vi "Teleop.vi"(10 "Match Info":T1={"Autonomous Elapsed Seconds"=0.0, "TeleOp Elapsed Seconds"=0.0, "Disabled Elapsed Seconds"=0.0, "Visited Autonomous"=FALSE, "Visited TeleOp"=FALSE, "Visited Disabled"=FALSE, "Autonomous Settings"={"Autonomous Style"=enum."Independent", "VI Refnum"=refnum}}, 11 "Call Context":T2) -> ()   [LabVIEW 2015]
doc: "This VI is called for each TeleOp packet received from the DS where the robot is not disabled. It is often used to read from the joysticks and update I/O or to update setpoints for timed control loops. It should complete and return within 20 milliseconds or it may miss DS packets."
uses:
  <vilib>/Rock Robotics/WPI/DriverStation/WPI_DriverStationDerivedRobotMode.ctl
  <vilib>/Rock Robotics/WPI/DriverStation/WPI_DriverStationMatch Info.ctl
  <vilib>/Rock Robotics/WPI/Solenoid/WPI_SolenoidValue.ctl
  <vilib>/Rock Robotics/WPI/Utilities/WPI_GetSetVariantRefNum.vi
  <vilib>/Rock Robotics/Network Tables/NT Read Boolean.vi
  <vilib>/Rock Robotics/Network Tables/NT Read Number.vi
  <vilib>/Rock Robotics/WPI/Solenoid/WPI_SolenoidSetEnum.vi
  <vilib>/addons/control/pid/NI_PID_pid.lvlib
  <vilib>/addons/control/pid/pid.llb/PID (DBL).vi
panel:
  out "Encodeur gauche max":dbl
  out "Encodeur droit max":dbl
  out "Encodeur gauche min":dbl
  out "Encodeur droit min":dbl
  out "Sample Slider 0":dbl(slide) scale=0.0..5.0
  out "Sample Boolean 1":bool
  out "Sample Boolean 0":bool
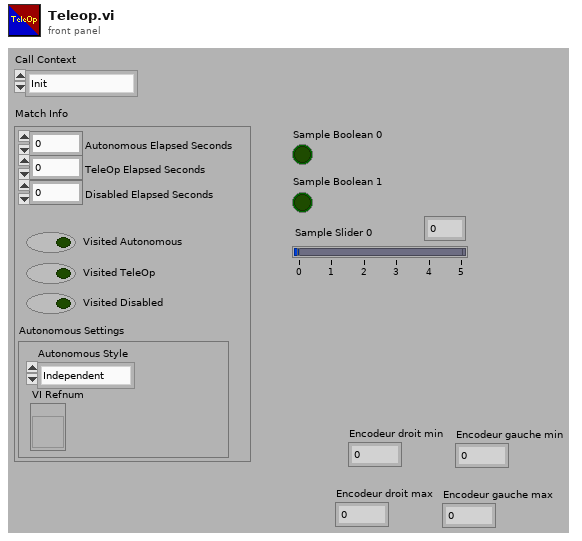
[diagram p1: front panel]
types:
  T1 = typedef "WPI_DriverStationMatch Info.ctl" = cluster{"Autonomous Elapsed Seconds":dbl, "TeleOp Elapsed Seconds":dbl, "Disabled Elapsed Seconds":dbl, "Visited Autonomous":bool, "Visited TeleOp":bool, "Visited Disabled":bool, "Autonomous Settings":cluster{"Autonomous Style":enum16{"Iterative", "Independent"}, "VI Refnum":refnum<vi>}}
  T2 = typedef "WPI_DriverStationDerivedRobotMode.ctl" = enum16{"Init", "Execute", "Stop"}
  T3 = typedef "WPI_JoystickDevRef.ctl" = cluster{"Device":T4}
  T4 = typedef "WPI_JoystickDeviceEnum.ctl" = enum16{"USB 0", "USB 1", "USB 2", "USB 3", "USB 4", "USB 5"}
  T5 = typedef "WPI_EncoderDevRef.ctl" = cluster{"DevStatus":errorcluster, "EncoderIndex":T6, "CounterIndex":T7, "DistancePerCount":dbl, "Decoding Type":T8}
  T6 = typedef "FPGA_EncoderIdx.ctl" = enum8{"Enc 0", "Enc 1", "Enc 2", "Enc 3", "Enc 4", "Enc 5", "Enc 6", "Enc 7", "Invalid"}
  T7 = typedef "FPGA_CounterCtrSystemIndex.ctl" = enum8{"Ctr 0", "Ctr 1", "Ctr 2", "Ctr 3", "Ctr 4", "Ctr 5", "Ctr 6", "Ctr 7", "Invalid"}
  T8 = typedef "WPI_EncoderType.ctl" = enum16{"1x", "2x", "4x"}
  T9 = cluster{"Buttons[0]":bool, "Buttons[1]":bool, "Buttons[2]":bool, "Buttons[3]":bool, "Buttons[4]":bool, "Buttons[5]":bool, "Buttons[6]":bool, "Buttons[7]":bool, "Buttons[8]":bool}
  T10 = cluster{"Axes[0]":dbl, "Axes[1]":dbl, "Axes[2]":dbl, "Axes[3]":dbl, "Axes[4]":dbl, "Axes[5]":dbl, "Axes[6]":dbl, "Axes[7]":dbl, "Axes[8]":dbl}
  T11 = cluster{"proportional gain (Kc)":dbl, "integral time (Ti, min)":dbl, "derivative time (Td, min)":dbl}
  T12 = typedef "WPI_MotorControlDeviceRef.ctl" = cluster{"DeviceStatus":errorcluster, "Type":T13, "PWM":cluster{"PWM Channel":T14, "DeadBand":T15}, "CAN":cluster{"Device Number":u8, "Control Mode":T16, "Semaphore":T17, "Max Vout":dbl, "TalonSRX Control Mode":T18}, "Invert":bool}
  T13 = typedef "WPI_MotorControlType.ctl" = enum16{"PWM", "CAN", "CANTalonSRX"}
  T14 = typedef "FPGA_DIOPWMChannel.ctl" = enum8{"PWM 0", "PWM 1", "PWM 2", "PWM 3", "PWM 4", "PWM 5", "PWM 6", "PWM 7", "PWM 8", "PWM 9", "PWM MXP 0", "PWM MXP 1", "PWM MXP 2", "PWM MXP 3", "PWM MXP 4", "PWM MXP 5", "PWM MXP 6", "PWM MXP 7", "PWM MXP 8", "PWM MXP 9", "Invalid"}
  T15 = typedef "WPI_PWMDeadband.ctl" = cluster{"Name":string, "maxPositivePwm":i32, "minPositivePwm":i32, "centerPwm":i32, "maxNegativePwm":i32, "minNegativePwm":i32, "angularRange":u16}
  T16 = typedef "WPI_CANJaguar_ControlMode.ctl" = enum8{"Percent VBus", "Current", "Speed", "Position", "Voltage"}
  T17 = typedef "Semaphore RefNum" = refnum<k1>
  T18 = typedef "WPI_CANTalonSRX_APIControlMode.ctl" = enum8{"Percent VBus", "Speed", "Position", "Slave", "Unchanged / Invalid", "Voltage Compensation", "Current", "Motion Profile"}
  T19 = typedef "WPI_SolenoidDevRef.ctl" = cluster{"DevStatus":errorcluster, "Pneumatics Control Module":u8, "Forward Solenoid Channel":T20, "Reverse Solenoid Channel":T20}
  T20 = typedef "WPI_SolenoidChannel.ctl" = enum8{"Solenoid 0", "Solenoid 1", "Solenoid 2", "Solenoid 3", "Solenoid 4", "Solenoid 5", "Solenoid 6", "Solenoid 7", "Invalid"}
  T21 = typedef "WPI_SolenoidValue.ctl" = enum16{"Off", "On", "Forward", "Reverse"}
  T22 = typedef "WPI_ServoDeviceRef.ctl" = cluster{"DeviceStatus":errorcluster, "PWM Channel":T14, "DeadBand":T15}
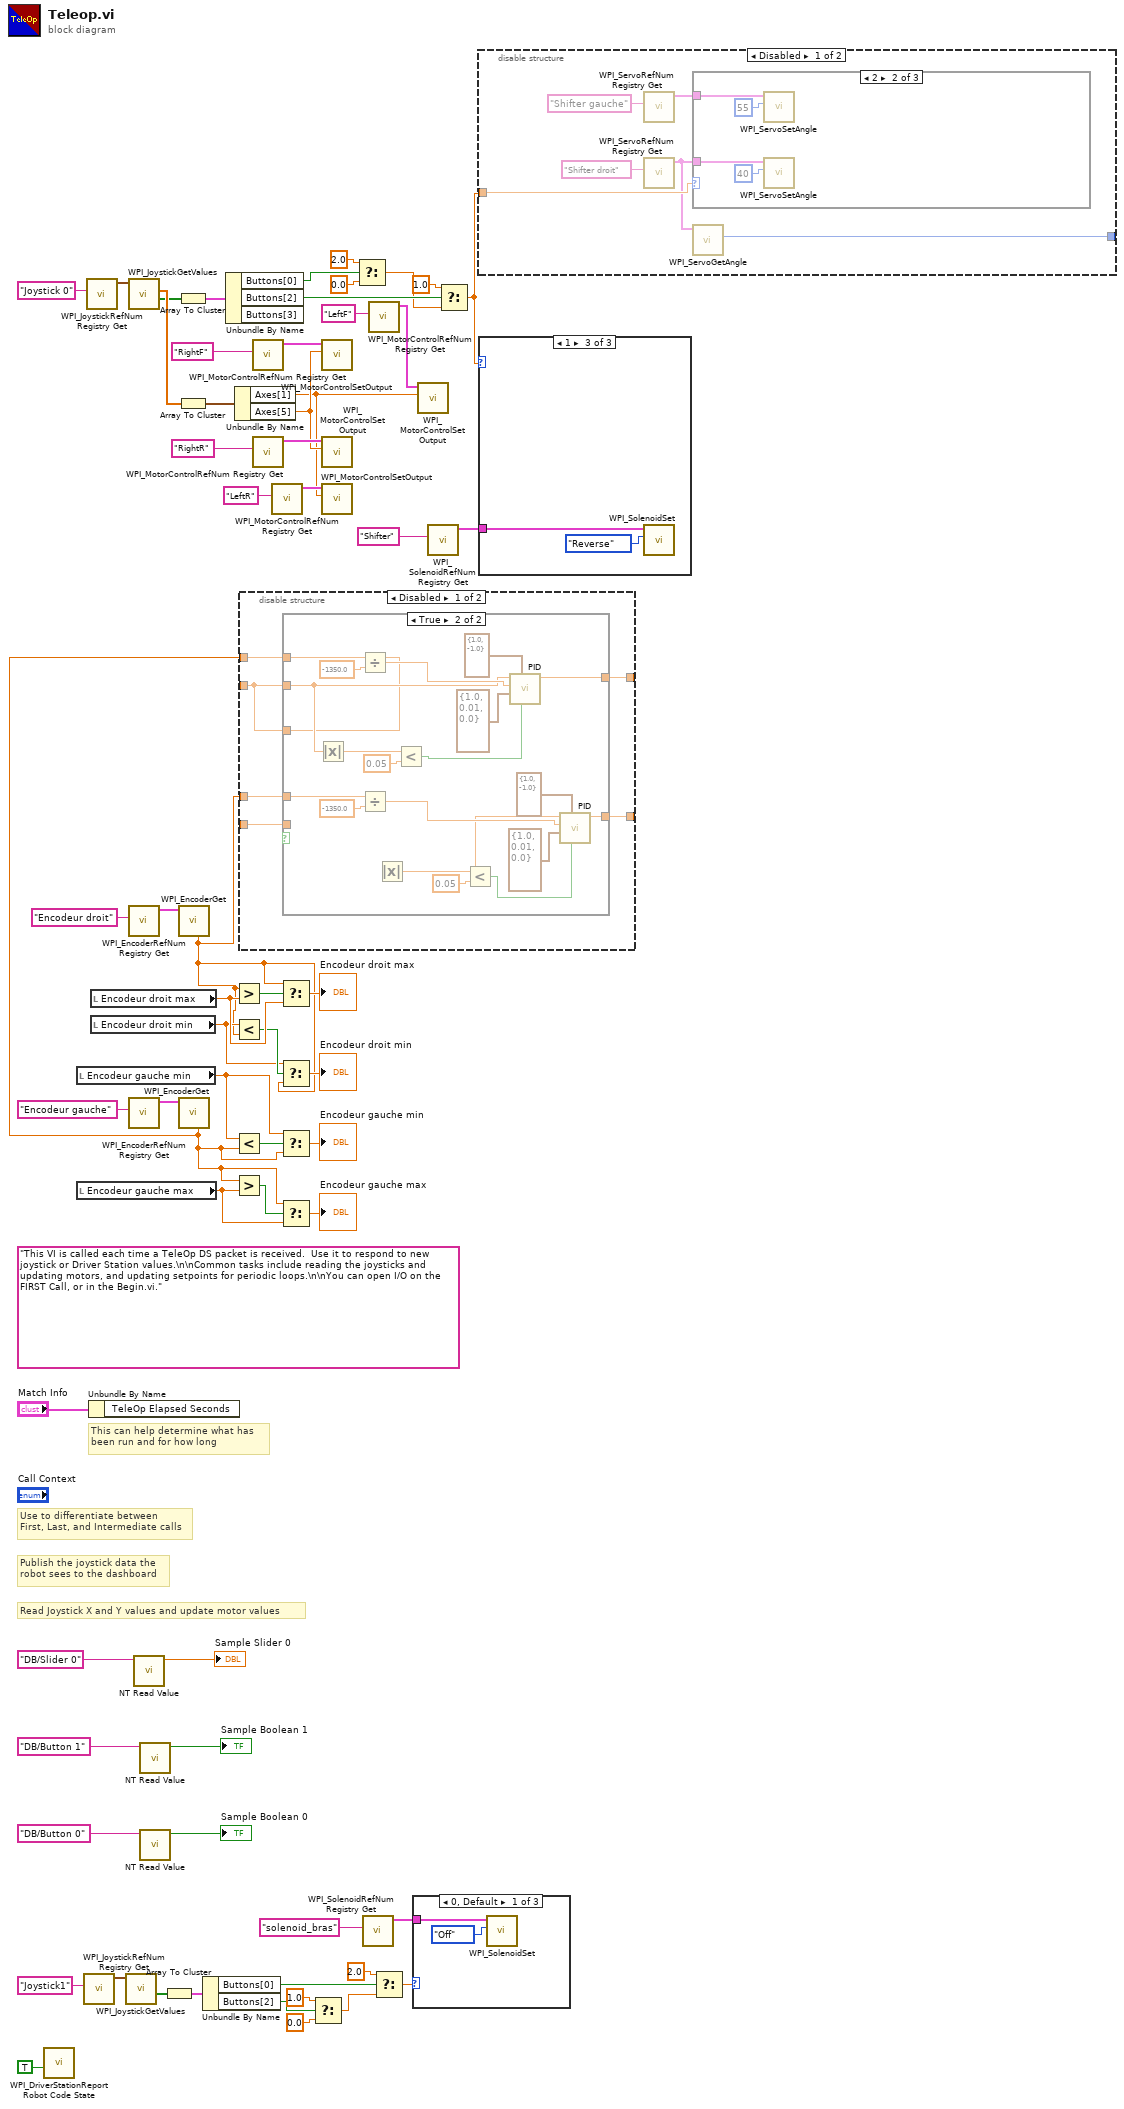
[diagram p0: block diagram]
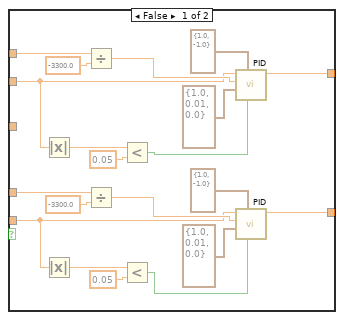
[diagram p2: hidden frame]
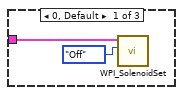
[diagram p4: hidden frame]
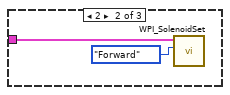
[diagram p5: hidden frame]
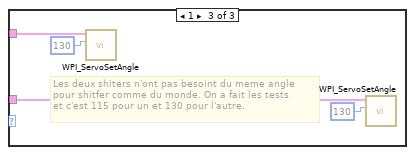
[diagram p7: hidden frame]
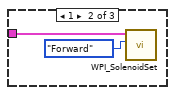
[diagram p9: hidden frame]
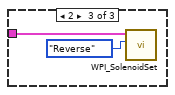
[diagram p10: hidden frame]
diagram:
  (unwired) "This VI is called each time a TeleOp DS packet is received.  Use it to respond to new joystick or Driver Station values.\n\nCommon tasks include reading the joysticks and updating motors, and updating setpoints for periodic loops.\n\nYou can open I/O on the FIRST Call, or in the Begin.vi."
  # "Publish the joystick data the\nrobot sees to the dashboard"
  # "Use to differentiate between\nFirst, Last, and Intermediate calls"
  # "This can help determine what has\nbeen run and for how long"
  # "Read Joystick X and Y values and update motor values"
  n1 = call <vilib>:"WPI_DriverStationReport Robot Code State.vi"("TeleOp"=TRUE ("Autonomous")) -> ()  [unwired: 10 in, 1 out]
  n2 = local read "Encodeur gauche min"() -> (w23:dbl)
  n3 = local read "Encodeur gauche max"() -> (w26:dbl)
  n4 = call <vilib>:"WPI_JoystickRefNum Registry Get.vi"("refnum name"="Joystick1") -> ("JoystickDevRef"=w43:T3)  [unwired: 1 in, 9 out]
  n5 = call <vilib>:"WPI_JoystickRefNum Registry Get.vi"("refnum name"="Joystick 0") -> ("JoystickDevRef"=w62:T3)  [unwired: 1 in, 9 out]
  n6 = Unbundle By Name("Match Info") -> ()  [unwired: 1 out]
  n7 = local read "Encodeur droit max"() -> (w21:dbl)
  n8 = local read "Encodeur droit min"() -> (w19:dbl)
  n9 = call <vilib>:"WPI_JoystickGetValues.vi"("JoystickDevRef"=w43) -> ("Buttons"=w44:bool[])  [unwired: 6 in, 4 out]
  n10 = call <vilib>:"WPI_JoystickGetValues.vi"("JoystickDevRef"=w62) -> ("Buttons"=w54:bool[], "Axes"=w56:dbl[])  [unwired: 6 in, 3 out]
  n11 = call <vilib>:"WPI_EncoderRefNum Registry Get.vi"("refnum name"="Encodeur droit") -> ("EncoderDevRef"=w30:T5)  [unwired: 9 in, 1 out]
  n12 = call <vilib>:"WPI_EncoderRefNum Registry Get.vi"("refnum name"="Encodeur gauche") -> ("EncoderDevRef"=w29:T5)  [unwired: 9 in, 1 out]
  n13 = call-poly <vilib>:"NT Read Value.vi"("Name"="DB/Slider 0" ("refnum name")) -> ("Numeric"=→"Sample Slider 0":dbl)  [unwired: 9 in, 1 out]
  n14 = call-poly <vilib>:"NT Read Value.vi"("Name"="DB/Button 1" ("refnum name")) -> ("Boolean"=→"Sample Boolean 1":bool)  [unwired: 9 in, 1 out]
  n15 = call-poly <vilib>:"NT Read Value.vi"("Name"="DB/Button 0" ("refnum name")) -> ("Boolean"=→"Sample Boolean 0":bool)  [unwired: 9 in, 1 out]
  n16 = Array To Cluster(array=w44) -> (cluster=w45:T9)
  n17 = Array To Cluster(array=w54) -> (cluster=w53:T9)
  n18 = Array To Cluster(array=w56) -> (cluster=w55:T10)
  n19 = call <vilib>:"WPI_EncoderGet.vi"("EncoderDevRef"=w30) -> ("Rate"=w7:dbl)  [unwired: 5 in, 5 out]
  n20 = call <vilib>:"WPI_EncoderGet.vi"("EncoderDevRef"=w29) -> ("Rate"=w8:dbl)  [unwired: 5 in, 5 out]
  n21 = Unbundle By Name(w45) -> ("Buttons[0]"=w38:bool, "Buttons[2]"=w37:bool)
  n22 = Unbundle By Name(w53) -> ("Buttons[0]"=w52:bool, "Buttons[2]"=w49:bool)  [unwired: 1 out]
  n23 = Greater?(x=w7, y=w21) -> (0:w22:bool)
  n24 = Less?(x=w19, y=w7) -> (x < y?=w20:bool)
  n25 = Less?(x=w23, y=w8) -> (x < y?=w24:bool)
  n26 = Greater?(x=w8, y=w26) -> (0:w27:bool)
  n27 = Unbundle By Name(w55) -> ("Axes[1]"=w1:dbl, "Axes[5]"=w2:dbl)
  n28 = disable-structure shown="Disabled" {
    disable-tunnel: w8 -> [w66 _]
    disable-tunnel: [w70 _] -> _
    disable-tunnel: [w65 _] -> _
    disable-tunnel: _ -> [w69 _]
    disable-tunnel: w7 -> [w68 _]
    disable-tunnel: [w67 _] -> _
    frame Disabled {
      n29 = case shown="True" {
        selector: _ -> [_ _]
        tunnel: w65 -> [w72 w102]
        tunnel: [w76 w103] -> w70
        tunnel: w69 -> [w71 _]
        tunnel: w68 -> [w73 w94]
        tunnel: [w75 w93] -> w67
        tunnel: w66 -> [w74 w91]
        tunnel: [_ w91] -> w65
        frame False {
          n30 = Absolute Value(x=w72) -> (abs(x)=w89:dbl)
          n31 = Absolute Value(x=w71) -> (abs(x)=w82:dbl)
          n32 = Divide(x=w74, y=-3300.0) -> (x/y=w87:dbl)
          n33 = Divide(x=w73, y=-3300.0) -> (x/y=w80:dbl)
          n34 = Less?(x=w89, y=0.05) -> (x < y?=w77:bool)
          n35 = Less?(x=w82, y=0.05) -> (x < y?=w84:bool)
          n36 = call-poly <vilib>:"PID.vi"("reinitialize? (F)"=w77, "output range"=cluster{"output high":dbl, "output low":dbl} {"output high"=1.0, "output low"=-1.0}, "PID gains"=T11 {"proportional gain (Kc)"=1.0, "integral time (Ti, min)"=0.01, "derivative time (Td, min)"=0.0}, "process variable"=w87, "setpoint"=w72) -> ("output"=w76:dbl)  [unwired: 5 in, 1 out]
          n37 = call-poly <vilib>:"PID.vi"("reinitialize? (F)"=w84, "output range"=cluster{"output high":dbl, "output low":dbl} {"output high"=1.0, "output low"=-1.0}, "PID gains"=T11 {"proportional gain (Kc)"=1.0, "integral time (Ti, min)"=0.01, "derivative time (Td, min)"=0.0}, "process variable"=w80, "setpoint"=w71) -> ("output"=w75:dbl)  [unwired: 5 in, 1 out]
        }
        frame True {
          n38 = Absolute Value(x=w102) -> (abs(x)=w108:dbl)
          n39 = Divide(x=w91, y=-1350.0) -> (x/y=w106:dbl)
          n40 = Divide(x=w94, y=-1350.0) -> (x/y=w97:dbl)
          n41 = Less?(x=w108, y=0.05) -> (x < y?=w110:bool)
          n42 = call-poly <vilib>:"PID.vi"("reinitialize? (F)"=w110, "output range"=cluster{"output high":dbl, "output low":dbl} {"output high"=1.0, "output low"=-1.0}, "PID gains"=T11 {"proportional gain (Kc)"=1.0, "integral time (Ti, min)"=0.01, "derivative time (Td, min)"=0.0}, "process variable"=w106, "setpoint"=w102) -> ("output"=w103:dbl)  [unwired: 5 in, 1 out]
          n43 = Absolute Value(x=w92) -> (abs(x)=w99:dbl)
          n44 = Less?(x=w99, y=0.05) -> (x < y?=w101:bool)
          n45 = call-poly <vilib>:"PID.vi"("reinitialize? (F)"=w101, "output range"=cluster{"output high":dbl, "output low":dbl} {"output high"=1.0, "output low"=-1.0}, "PID gains"=T11 {"proportional gain (Kc)"=1.0, "integral time (Ti, min)"=0.01, "derivative time (Td, min)"=0.0}, "process variable"=w97) -> ("output"=w93:dbl, "setpoint"=w92:dbl)  [unwired: 5 in, 1 out]
        }
      }
    }
    frame Enabled {
    }
  }
  n46 = call <vilib>:"WPI_MotorControlRefNum Registry Get.vi"("refnum name"="RightF") -> ("MotorControlDevRef"=w14:T12)  [unwired: 9 in, 1 out]
  n47 = call <vilib>:"WPI_MotorControlRefNum Registry Get.vi"("refnum name"="RightR") -> ("MotorControlDevRef"=w13:T12)  [unwired: 9 in, 1 out]
  n48 = call <vilib>:"WPI_MotorControlRefNum Registry Get.vi"("refnum name"="LeftR") -> ("MotorControlDevRef"=w15:T12)  [unwired: 9 in, 1 out]
  n49 = Select(t=w7, s=w22, f=w21) -> (s? t:f=→"Encodeur droit max":dbl)
  n50 = Select(t=w19, s=w20, f=w7) -> (s? t:f=→"Encodeur droit min":dbl)
  n51 = Select(t=w23, s=w24, f=w8) -> (s? t:f=→"Encodeur gauche min":dbl)
  n52 = Select(t=w8, s=w27, f=w26) -> (s? t:f=→"Encodeur gauche max":dbl)
  n53 = Select(t=1.0, s=w37, f=0.0) -> (s? t:f=w39:dbl)
  n54 = call <vilib>:"WPI_MotorControlSetOutput.vi"("Output"=w2, "MotorControlDevRef"=w14) -> ()  [unwired: 7 in, 3 out]
  n55 = call <vilib>:"WPI_MotorControlSetOutput.vi"("Output"=w2, "MotorControlDevRef"=w13) -> ()  [unwired: 7 in, 3 out]
  n56 = call <vilib>:"WPI_MotorControlSetOutput.vi"("Output"=w1, "MotorControlDevRef"=w15) -> ()  [unwired: 7 in, 3 out]
  n57 = Select(t=2.0, s=w52, f=0.0) -> (s? t:f=w48:dbl)
  n58 = call <vilib>:"WPI_SolenoidRefNum Registry Get.vi"("refnum name"="solenoid_bras") -> ("SolenoidDevRef"=w32:T19)  [unwired: 9 in, 1 out]
  n59 = call <vilib>:"WPI_MotorControlRefNum Registry Get.vi"("refnum name"="LeftF") -> ("MotorControlDevRef"=w16:T12)  [unwired: 9 in, 1 out]
  n60 = Select(t=2.0, s=w38, f=w39) -> (s? t:f=w33:dbl)
  n61 = case shown="0, Default" w33 {
    tunnel: w32 -> [w111 w114 w115]
    frame 0, Default {
      n62 = call-poly <vilib>:"WPI_SolenoidSet.vi"("Value"=WPI_SolenoidValue."Off", "SolenoidDevRef"=w111) -> ()  [unwired: 8 in, 2 out]
    }
    frame 1 {
      n63 = call-poly <vilib>:"WPI_SolenoidSet.vi"("Value"=WPI_SolenoidValue."Forward", "SolenoidDevRef"=w114) -> ()  [unwired: 8 in, 2 out]
    }
    frame 2 {
      n64 = call-poly <vilib>:"WPI_SolenoidSet.vi"("Value"=WPI_SolenoidValue."Reverse", "SolenoidDevRef"=w115) -> ()  [unwired: 8 in, 2 out]
    }
  }
  n65 = call <vilib>:"WPI_MotorControlSetOutput.vi"("Output"=w1, "MotorControlDevRef"=w16) -> ()  [unwired: 7 in, 3 out]
  n66 = call <vilib>:"WPI_SolenoidRefNum Registry Get.vi"("refnum name"="Shifter") -> ("SolenoidDevRef"=w5:T19)  [unwired: 9 in, 1 out]
  n67 = Select(t=1.0, s=w49, f=w48) -> (s? t:f=w4:dbl)
  n68 = disable-structure shown="Disabled" {
    disable-tunnel: w4 -> [w119 _]
    disable-tunnel: [w117 _] -> _
    frame Disabled {
      n69 = call <vilib>:"WPI_ServoRefNum Registry Get.vi"("refnum name"="Shifter gauche") -> ("ServoDeviceRef"=w120:T22)  [unwired: 9 in, 1 out]
      n70 = call <vilib>:"WPI_ServoRefNum Registry Get.vi"("refnum name"="Shifter droit") -> ("ServoDeviceRef"=w118:T22)  [unwired: 9 in, 1 out]
      n71 = case shown="2" w119 {
        tunnel: w120 -> [_ w126 w130]
        tunnel: w118 -> [_ w125 w129]
        frame 0, Default {
        }
        frame 2 {
          n72 = call <vilib>:"WPI_ServoSetAngle.vi"("Angle"=55, "ServoDeviceRef"=w126) -> ()  [unwired: 8 in, 2 out]
          n73 = call <vilib>:"WPI_ServoSetAngle.vi"("Angle"=40, "ServoDeviceRef"=w125) -> ()  [unwired: 8 in, 2 out]
        }
        frame 1 {
          # "Les deux shiters n'ont pas besoint du meme angle \npour shitfer comme du monde. On a fait les tests \net c'est 115 pour un et 130 pour l'autre."
          n74 = call <vilib>:"WPI_ServoSetAngle.vi"("Angle"=130, "ServoDeviceRef"=w130) -> ()  [unwired: 8 in, 2 out]
          n75 = call <vilib>:"WPI_ServoSetAngle.vi"("Angle"=130, "ServoDeviceRef"=w129) -> ()  [unwired: 8 in, 2 out]
        }
      }
      n76 = call <vilib>:"WPI_ServoGetAngle.vi"("ServoDeviceRef"=w118) -> ("Angle"=w117:u16)  [unwired: 7 in, 2 out]
    }
    frame Enabled {
    }
  }
  n77 = case shown="1" w4 {
    tunnel: w5 -> [w132 w134 w135]
    frame 0, Default {
      n78 = call-poly <vilib>:"WPI_SolenoidSet.vi"("Value"=WPI_SolenoidValue."Off", "SolenoidDevRef"=w132) -> ()  [unwired: 8 in, 2 out]
    }
    frame 2 {
      n79 = call-poly <vilib>:"WPI_SolenoidSet.vi"("Value"=WPI_SolenoidValue."Forward", "SolenoidDevRef"=w134) -> ()  [unwired: 8 in, 2 out]
    }
    frame 1 {
      n80 = call-poly <vilib>:"WPI_SolenoidSet.vi"("Value"=WPI_SolenoidValue."Reverse", "SolenoidDevRef"=w135) -> ()  [unwired: 8 in, 2 out]
    }
  }
